vi "Advanced OM Config.vi"(8 "error in (no error)":errorcluster, 11 "OM  Location":T3) -> (0 "error out":errorcluster)   [LabVIEW 2013]
uses:
  lib/Data Access Objects/Metadata/LBCB Location.ctl
  lib/Data Access Objects/Application/Number Of LBCBs.ctl
  lib/Apps/Yes No Button.ctl
  lib/Data Access Objects/Metadata/Persistant DAO Actions.ctl
panel:
  in  "Ok":bool
  in  "Rigid Connection":T1
  in  "Number of LBCBs":T2
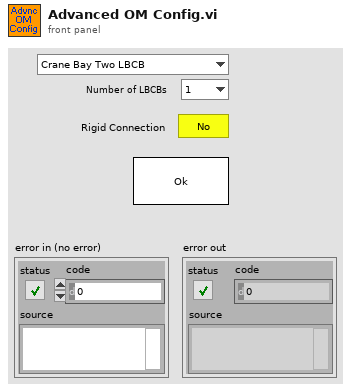
[diagram p1: front panel]
types:
  T1 = typedef "Yes No Button.ctl" = bool
  T2 = typedef "Number Of LBCBs.ctl" = enum16{"1", "2"}
  T3 = typedef "LBCB Location.ctl" = enum16{"Crane Bay Two LBCB", "Crane Bay One LBCB", "5th Scale Two LBCB", "5th Scale One LBCB", "Portable LBCB", "University of Houston LBCB"}
  T4 = typedef "Persistant DAO Actions.ctl" = enum16{"Init", "Get", "Set", "Load", "Save"}
  T5 = typedef "Timing & Logging Parameters.ctl" = cluster{"Monitor Loop":T6, "Ramp Time":T6, "Log Loop":T6, "TCP to DAQ":T6, "Logging Directory":path, "Log File Size (MBytes)":i64, "Volt Logging Loop":T6, "2 LBCB Archiving Mode":bool, "Fake":bool}
  T6 = typedef "Timing Parameters.ctl" = cluster{"Interval":dbl, "Rate ":dbl}
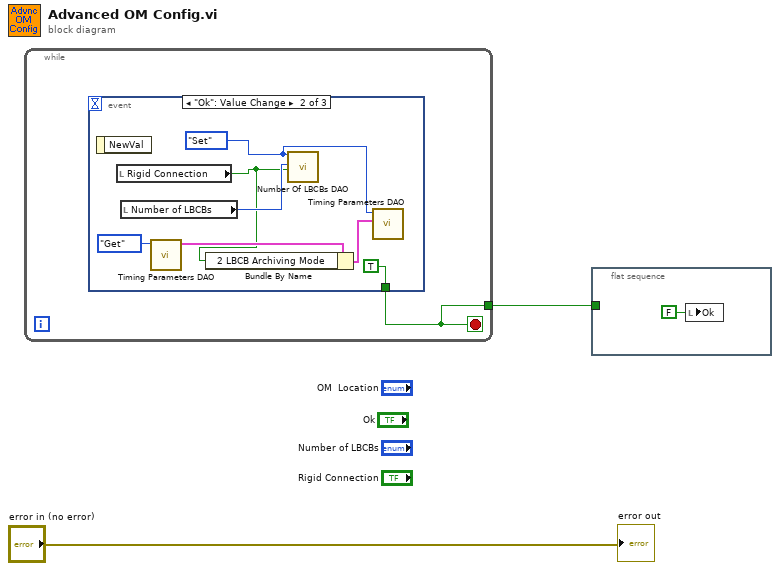
[diagram p0: block diagram]
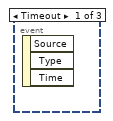
[diagram p2: hidden frame]
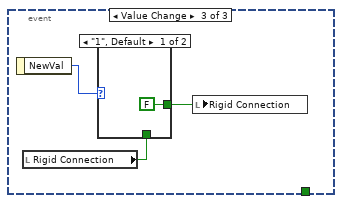
[diagram p3: hidden frame]
diagram:
  n1 = while {
    tunnel: [w3] -> w2
    stop <- w3 stop-if-true
    n2 = event shown="[1] \"Ok\": Value Change" {
      selector: _ -> [_ _ _]
      dyn-events: _ -> [_ _ _]
      timeout: _ -> [_ _ _]
      tunnel: [_ TRUE _] -> w3
      event Timeout {
        n3 = event-data() -> ()  [unwired: 1 in, 3 out]
      }
      event "Ok": Value Change {
        w5 = Persistant_DAO_Actions."Set" ("Actions")
        n4 = event-data() -> ()  [unwired: 1 in, 1 out]
        n5 = local read "Rigid Connection"() -> (w4:T1)
        n6 = local read "Number of LBCBs"() -> (w9:T2)
        n7 = call "Timing Parameters DAO.vi"("Actions"=Persistant_DAO_Actions."Get") -> ("Application Timing and Logging Out"=w7:T5)  [unwired: 8 in, 2 out]
        n8 = Bundle By Name(cluster=w7, "2 LBCB Archiving Mode"=w4) -> (w6:T5)
        n9 = call "Number Of LBCBs DAO.vi"("Actions"=w5, "Number of\nLBCBs In"=w9, "Rigid Connection In"=w4) -> ()  [unwired: 11 in, 6 out]
        n10 = call "Timing Parameters DAO.vi"("Application Timing and Logging In"=w6, "Actions"=w5) -> ()  [unwired: 7 in, 3 out]
      }
      event Value Change {
        n11 = event-data() -> ("NewVal"=w13:T2)  [unwired: 1 in]
        n12 = local read "Rigid Connection"() -> (w12:T1)
        n13 = case shown="\"1\", Default" w13 {
          tunnel: w12 -> [_ w15]
          tunnel: [T1 FALSE ("Rigid Connection") w15] -> w11
          frame "1", Default {
          }
          frame "2" {
          }
        }
        n14 = local write "Rigid Connection"(w11) -> ()
      }
    }
  }
  n15 = flat-sequence {
    tunnel: w2 -> [_]
    frame #0 {
      n16 = local write "Ok"(FALSE ("Ok")) -> ()
    }
  }
  "error out" <- "error in (no error)"
